vi "总磷氨氮插入数据.vi"(0 "table":string, 5 "data":T2={"时间标识"=timestamp(0 s since 1904-01-01), "测量模式"=enum."水样测试", "数据标记表"="N", "监测值"=0.0, "单位"=0, "数据标识"="", "因子编码"=0, "标样参考值"=0.0, "F0"=0.0, "F1"=0.0, "F2"=0.0, "F3"=0.0, "F4"=0.0, "F5"=0.0, "F6"=0.0, "F7"=0.0, "X"=0.0, "温度"=0.0, "湿度"=0.0, "量程标识"="", "SN"="", "跨度值"=0.0, "X1"=0.0} {"单位" items=["μg/L", "mg/L", "ppm", "mg/m3", "cm", "ppb", "μg/m3", "%", "nmol/mol", "μmol/mol", "MPN/L", "MPN/100ml", "ng/m3", "NTU", "无量纲", "ms/cm", "μs/cm"]}, 7 "关键参数":T1, 11 "error in (no error)":errorcluster) -> (15 "error out":errorcluster)   [LabVIEW 2016, in "斯坦道总磷总氮.lvlib"]
uses:
  <vilib>/Utility/error.llb/DialogType.ctl
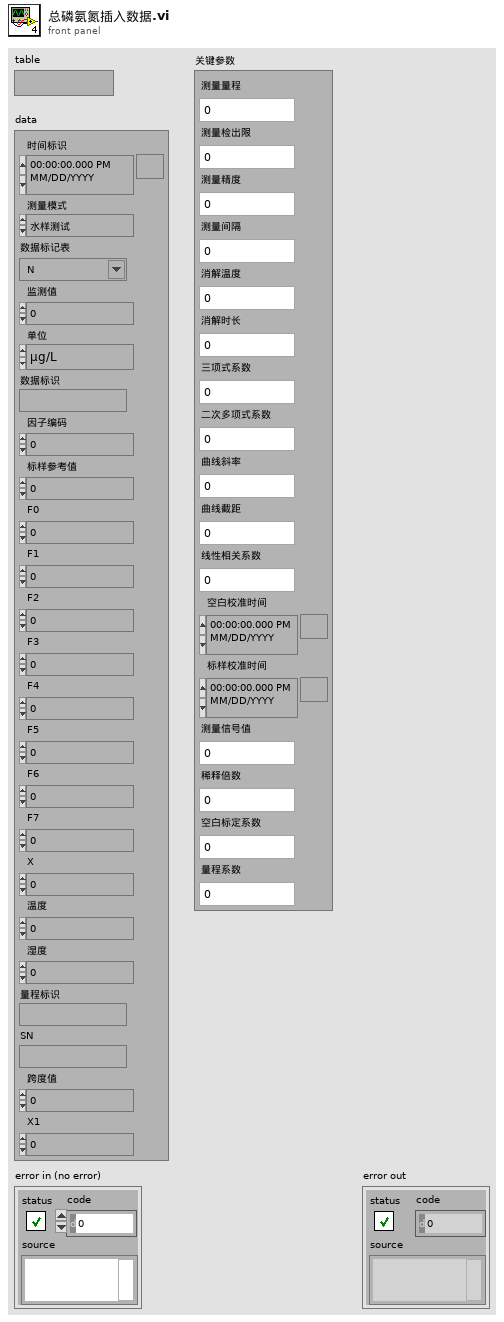
[diagram p1: front panel]
types:
  T1 = typedef "斯坦道总磷总氮.lvlib/关键参数.ctl" = cluster{"测量量程":sgl, "测量检出限":sgl, "测量精度":sgl, "测量间隔":sgl, "消解温度":sgl, "消解时长":sgl, "三项式系数":sgl, "二次多项式系数":sgl, "曲线斜率":sgl, "曲线截距":sgl, "线性相关系数":sgl, "空白校准时间":timestamp, "标样校准时间":timestamp, "测量信号值":sgl, "稀释倍数":sgl, "空白标定系数":sgl, "量程系数":sgl}
  T2 = cluster{"时间标识":timestamp, "测量模式":enum16{"维护数据", "水样测试", "标样核查", "零点核查", "跨度核查", "空白测试", "平行样测试", "加标回收", "空白校准", "标样校准", "初始化（清洗）", "快捷测试"}, "数据标记表":string, "监测值":sgl, "单位":u16, "数据标识":string, "因子编码":u32, "标样参考值":sgl, "F0":sgl, "F1":sgl, "F2":sgl, "F3":sgl, "F4":sgl, "F5":sgl, "F6":sgl, "F7":sgl, "X":sgl, "温度":sgl, "湿度":sgl, "量程标识":string, "SN":string, "跨度值":sgl, "X1":sgl}
  T3 = typedef "DialogType.ctl" = u16
  T4 = typedef "营养盐字段定义.ctl" = cluster{"时间":timestamp, "测量模式":string, "数据类型":string, "检测值":sgl, "单位":string, "数据标识":string, "X":sgl, "量程标识":string, "SN":string, "标样参考值":sgl, "跨度值":sgl, "F0":sgl, "F1":sgl, "F2":sgl, "F3":sgl, "F4":sgl, "F5":sgl, "F6":sgl, "F7":sgl, "X1":sgl, "因子编码":string, "温度":sgl, "湿度":sgl, "测量量程":sgl, "测量检出限":sgl, "测量精度":sgl, "测量间隔":sgl, "消解温度":sgl, "消解时长":sgl, "三项式系数":sgl, "二次多项式系数":sgl, "曲线斜率":sgl, "曲线截距":sgl, "线性相关系数":sgl, "空白校准时间":timestamp, "标样校准时间":timestamp, "测量信号值":sgl, "稀释倍数":sgl, "空白标定系数":sgl, "量程系数":sgl, "LastTime":timestamp}
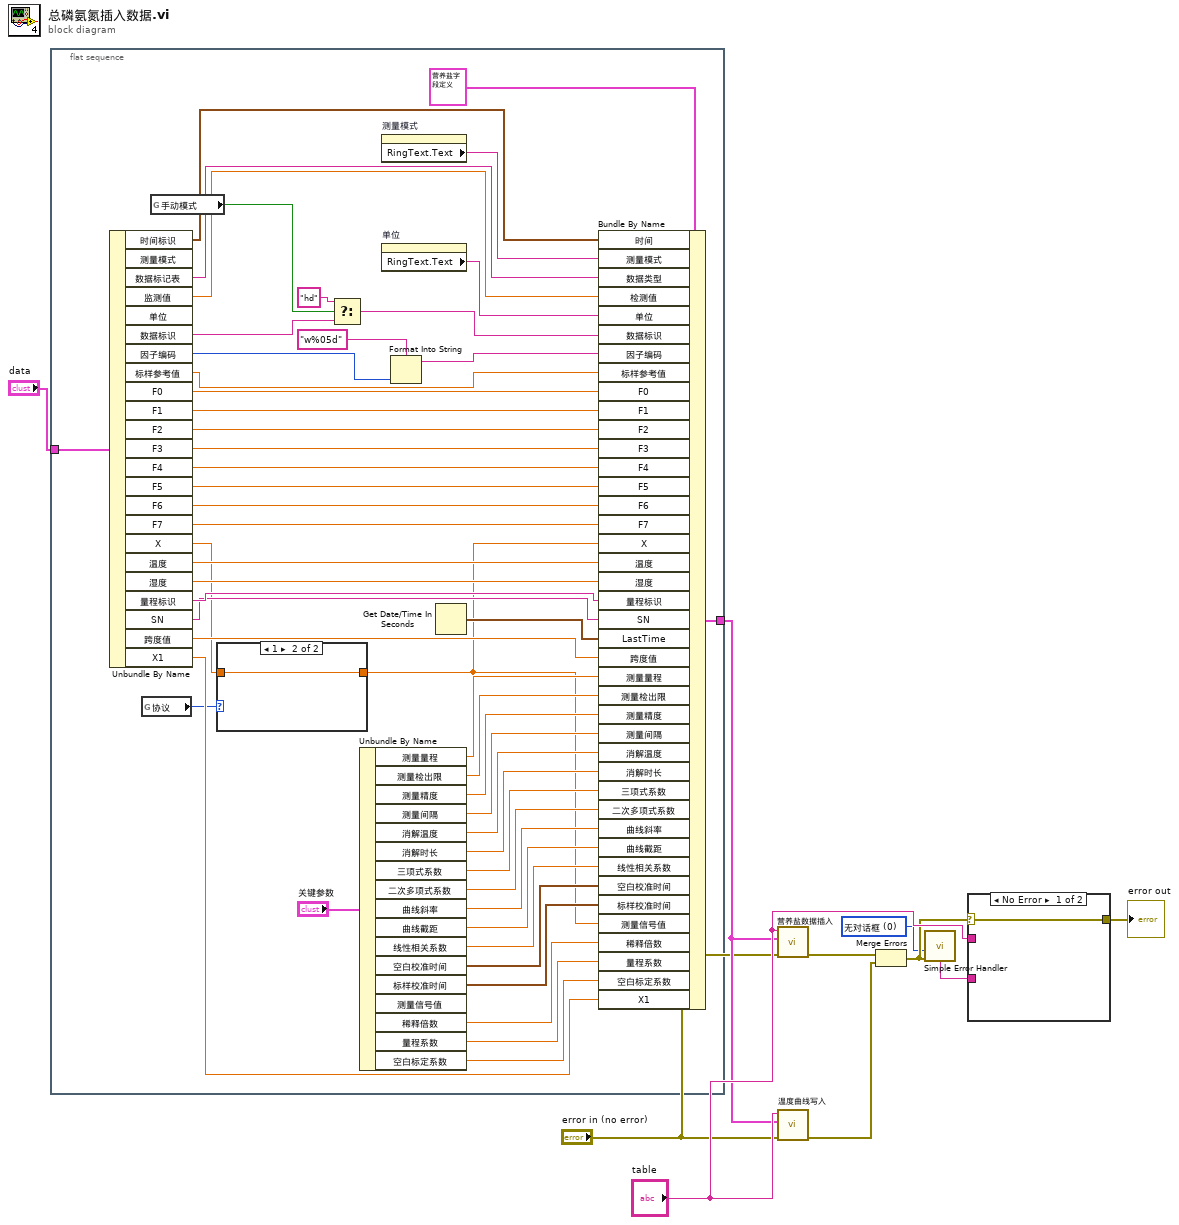
[diagram p0: block diagram]
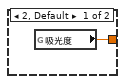
[diagram p2: hidden frame]
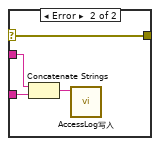
[diagram p3: hidden frame]
diagram:
  w2 = T3 0 items=["无对话框", "确定信息", "继续或停止信息", "确定信息＋警告", "继续/停止+警告"] ("type of dialog (OK msg:1)")
  n1 = flat-sequence {
    tunnel: "data" -> [w42]
    tunnel: [w18] -> w6
    frame #0 {
      n2 = Unbundle By Name(w42) -> ("时间标识"=w61:timestamp, "数据标记表"=w59:string, "监测值"=w58:sgl, "数据标识"=w15:string, "因子编码"=w41:u32, "标样参考值"=w56:sgl, "F0"=w55:sgl, "F1"=w54:sgl, "F2"=w53:sgl, "F3"=w52:sgl, "F4"=w51:sgl, "F5"=w50:sgl, "F6"=w49:sgl, "F7"=w48:sgl, "X"=w12:sgl, "温度"=w47:sgl, "湿度"=w46:sgl, "量程标识"=w45:string, "SN"=w44:string, "跨度值"=w38:sgl, "X1"=w20:sgl)  [unwired: 2 out]
      n3 = global read "总磷总氮断电保存全局变量.vi" "协议"() -> (w13:u16)
      n4 = global read "VAR总磷总氮全局变量.vi" "手动模式"() -> (w17:bool)
      n5 = case shown="1" w13 {
        tunnel: w12 -> [_ w63]
        tunnel: [w62 w63] -> w11
        frame 2, Default {
          n6 = global read "总磷总氮断电保存全局变量.vi" "吸光度"() -> (w62:sgl)
        }
        frame 1 {
        }
      }
      n7 = Select(t="hd", s=w17, f=w15) -> (s? t:f=w14:string)
      n8 = Unbundle By Name("关键参数") -> ("测量量程"=w36:sgl, "测量检出限"=w35:sgl, "测量精度"=w34:sgl, "测量间隔"=w33:sgl, "消解温度"=w32:sgl, "消解时长"=w31:sgl, "三项式系数"=w30:sgl, "二次多项式系数"=w29:sgl, "曲线斜率"=w28:sgl, "曲线截距"=w27:sgl, "线性相关系数"=w26:sgl, "空白校准时间"=w25:timestamp, "标样校准时间"=w24:timestamp, "稀释倍数"=w23:sgl, "量程系数"=w22:sgl, "空白标定系数"=w21:sgl)  [unwired: 1 out]
      n9 = property on="测量模式" class="Enum (strict)"() -> ("RingText.Text"=w60:string)  [unwired: 2 in, 2 out]
      n10 = property on="单位" class="Ring (strict)"() -> ("RingText.Text"=w57:string)  [unwired: 2 in, 2 out]
      n11 = Format Into String(format string="w%05d" ("格式字符串"), w41) -> (resulting string=w39:string)  [unwired: 2 in, 1 out]
      n12 = Get Date/Time In Seconds() -> (seconds since 1Jan1904=w43:timestamp)
      n13 = Bundle By Name(cluster=T4 {"时间"=timestamp(0 s since 1904-01-01), "测量模式"="水样测试", "数据类型"="N", "检测值"=0.0, "单位"="mg/L", "数据标识"="N", "X"=0.0, "量程标识"="", "SN"="", "标样参考值"=0.0, "跨度值"=0.0, "F0"=0.0, "F1"=0.0, "F2"=0.0, "F3"=0.0, "F4"=0.0, "F5"=0.0, "F6"=0.0, "F7"=0.0, "X1"=0.0, "因子编码"="", "温度"=0.0, "湿度"=0.0, "测量量程"=0.0, "测量检出限"=0.0, "测量精度"=0.0, "测量间隔"=0.0, "消解温度"=0.0, "消解时长"=0.0, "三项式系数"=0.0, "二次多项式系数"=0.0, "曲线斜率"=0.0, "曲线截距"=0.0, "线性相关系数"=0.0, "空白校准时间"=timestamp(0 s since 1904-01-01), "标样校准时间"=timestamp(0 s since 1904-01-01), "测量信号值"=0.0, "稀释倍数"=0.0, "空白标定系数"=0.0, "量程系数"=0.0, "LastTime"=timestamp(0 s since 1904-01-01)} ("data"), "时间"=w61, "测量模式"=w60, "数据类型"=w59, "检测值"=w58, "单位"=w57, "数据标识"=w14, "因子编码"=w39, "标样参考值"=w56, "F0"=w55, "F1"=w54, "F2"=w53, "F3"=w52, "F4"=w51, "F5"=w50, "F6"=w49, "F7"=w48, "X"=w11, "温度"=w47, "湿度"=w46, "量程标识"=w45, "SN"=w44, "LastTime"=w43, "跨度值"=w38, "测量量程"=w36, "测量检出限"=w35, "测量精度"=w34, "测量间隔"=w33, "消解温度"=w32, "消解时长"=w31, "三项式系数"=w30, "二次多项式系数"=w29, "曲线斜率"=w28, "曲线截距"=w27, "线性相关系数"=w26, "空白校准时间"=w25, "标样校准时间"=w24, "测量信号值"=w11, "稀释倍数"=w23, "量程系数"=w22, "空白标定系数"=w21, "X1"=w20) -> (w18:T4)
    }
  }
  n14 = call "营养盐数据插入.vi"("Tabe Name"="table", "data"=w6, "错误输入（无错误）"="error in (no error)") -> ("错误输出"=w8:errorcluster)  [unwired: 7 in]
  n15 = call "温度曲线写入.vi"("error in (no error)"="error in (no error)", "columns"=w6, "table"="table") -> ("错误输出"=w4:errorcluster)  [unwired: 8 in]
  n16 = Merge Errors(w8, w4) -> (w3:errorcluster)
  n17 = call <vilib>:"Simple Error Handler.vi"("type of dialog (OK msg:1)"=w2, "error in (no error)"=w3) -> ("message"=w1:string)  [unwired: 3 in, 4 out]
  n18 = case shown="No Error" w3 {
    selector: w3 -> [w64 w68]
    tunnel: [w64 w68] -> w10
    tunnel: "table" -> [_ w67]
    tunnel: w1 -> [_ w66]
    frame No Error {
    }
    frame Error {
      n19 = Concatenate Strings(w67, w66) -> (w65:string)
      n20 = call "AccessLog写入.vi"("Log"=w65) -> ()  [unwired: 11 in]
    }
  }
  "error out" <- w10
